vi "InvertOrientation.vi"(0 "object in":refnum<class "KickToSkill.lvclass">, 3 "orientation":dbl, 5 "error in (no error)":errorcluster) -> (14 "object out":refnum<class "KickToSkill.lvclass">, 17 "inverted":dbl, 19 "error out":errorcluster)   [LabVIEW 2023, in "KickToSkill.lvclass"]
uses:
  KickToSkill.lvclass
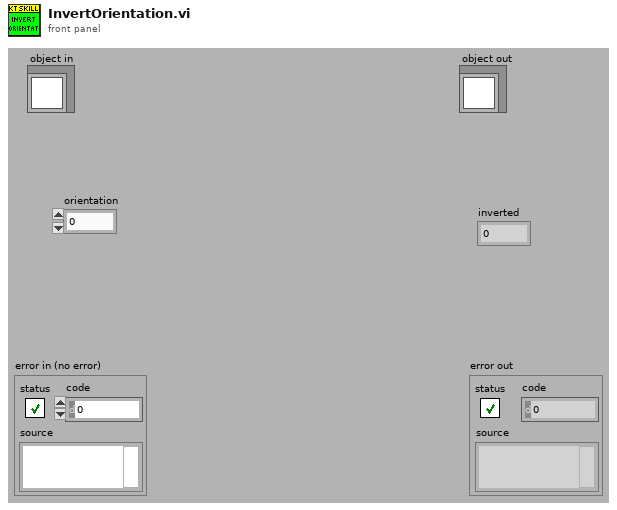
[diagram p1: front panel]
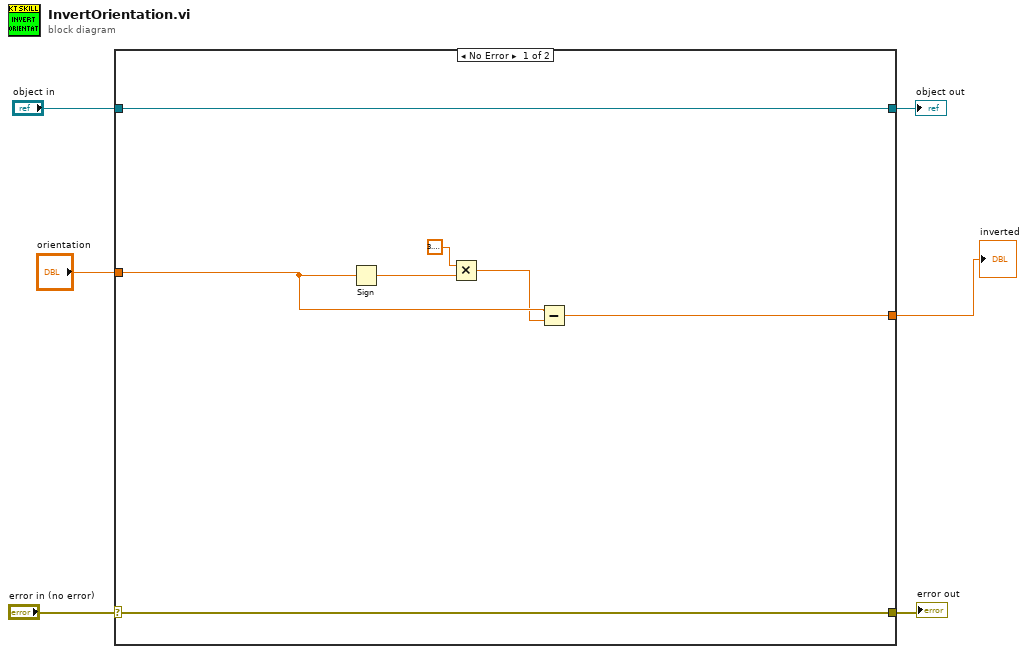
[diagram p0: block diagram]
diagram:
  n1 = case shown="No Error" "error in (no error)" {
    selector: "error in (no error)" -> [w13 w16]
    tunnel: [w13 w16] -> w5
    tunnel: [w12 w15] -> w3
    tunnel: "object in" -> [w12 w15]
    tunnel: "orientation" -> [w9 w14]
    tunnel: [w7 w14] -> w1
    frame No Error {
      n2 = Sign(1:w9) -> (0:w10:dbl)
      n3 = Multiply(x=3.141592653589793, y=w10) -> (x*y=w8:dbl)
      n4 = Subtract(x=w9, y=w8) -> (x-y=w7:dbl)
    }
    frame Error {
    }
  }
  "error out" <- w5
  "object out" <- w3
  "inverted" <- w1
